vi "Robot.Interface.Startup.vi"(8 "error in (no error)":errorcluster, 11 "Robot_Interface in":refnum<class "Robot_Interface.lvclass">) -> (0 "error out":errorcluster, 3 "Robot_Interface out":refnum<class "Robot_Interface.lvclass">)   [LabVIEW 2015, in "Robot_Interface.lvclass"]
uses:
  Robot_Interface.lvclass
  Robot_Interface.lvclass/Robot_Interface.ctl
  <vilib>/JKI/JKI SMO/SMO/SMO.lvclass
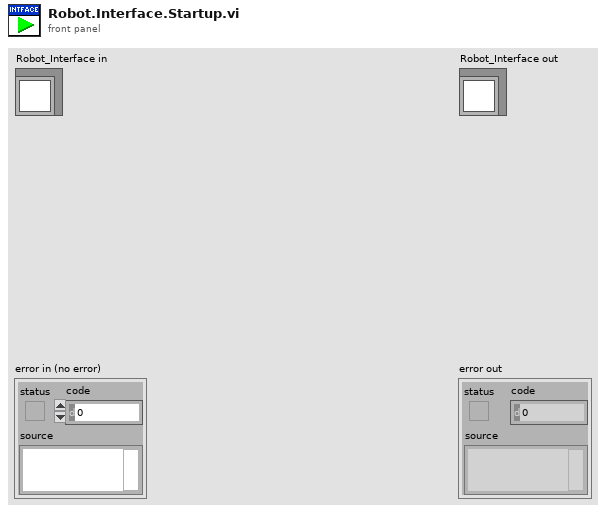
[diagram p1: front panel]
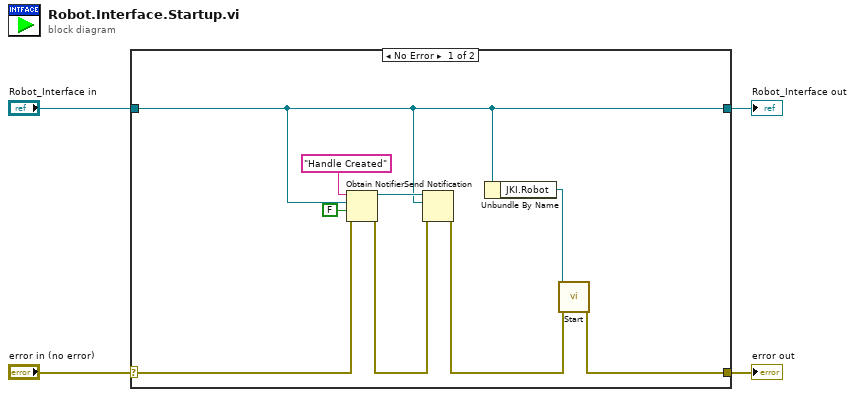
[diagram p0: block diagram]
diagram:
  n1 = case shown="No Error" "error in (no error)" {
    selector: "error in (no error)" -> [w10 w15]
    tunnel: [w5 w15] -> w3
    tunnel: [w8 w14] -> w1
    tunnel: "Robot_Interface in" -> [w8 w14]
    frame No Error {
      n2 = Obtain Notifier(name (unnamed)="Handle Created", notification data type=w8, create if not found? (T)=FALSE, error in (no error)=w10) -> (notifier out=w12:refnum<notifier>, error out=w9:errorcluster)  [unwired: 1 out]
      n3 = Send Notification(notification=w8, notifier=w12, error in (no error)=w9) -> (error out=w6:errorcluster)  [unwired: 1 out]
      n4 = Unbundle By Name(w8) -> ("JKI.Robot"=w7:refnum<class "JKI.Robot.SMO.Base.lvclass">)
      n5 = call <vilib>:"Start.vi"("error in (no error)"=w6, "SMO"=w7) -> ("error out"=w5:errorcluster)  [unwired: 8 in, 1 out]
    }
    frame Error {
    }
  }
  "error out" <- w3
  "Robot_Interface out" <- w1
